vi "PlayConvolution.vi"(11 "File":T1) -> ()   [LabVIEW 2022 SP3]
uses:
  Curtin1_Label.ctl
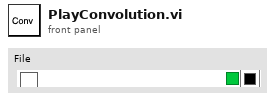
[diagram p1: front panel]
types:
  T1 = typedef "Curtin1_Label.ctl" = cluster{"Show?":bool, "Name":string, "Color":u32, "Path":path, "Show Notes":bool, "correlate":bool}
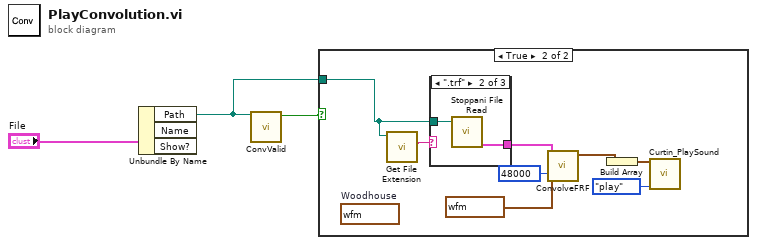
[diagram p0: block diagram]
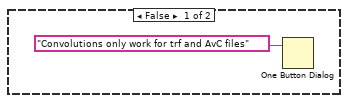
[diagram p2: hidden frame]
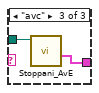
[diagram p4: hidden frame]
diagram:
  n1 = Unbundle By Name("File") -> ("Path"=w1:path)  [unwired: 2 out]
  n2 = call "ConvValid.vi"("Path"=w1) -> ("Valid"=w2:bool)  [unwired: 10 in]
  n3 = case shown="True" w2 {
    tunnel: w1 -> [_ w11]
    frame False {
      n4 = One Button Dialog(message="Convolutions only work for trf and AvC files" ("element")) -> ()  [unwired: 1 in, 1 out]
    }
    frame True {
      (unwired) waveform(dbl)[] [{"t0"=timestamp(0 s since 1904-01-01), "dt"=2.5e-05, "Y"=array[400000 elements]}]  # Woodhouse
      n5 = call <vilib>:"Get File Extension.vi"("file"=w11) -> ("lowercase file extension"=w12:string)  [unwired: 6 in, 4 out]
      n6 = case shown="\".trf\"" w12 {
        tunnel: [_ w14 w15] -> w10
        tunnel: w11 -> [_ w13 w16]
        frame Default {
        }
        frame ".trf" {
          n7 = call "Stoppani File Read.vi"("String in"=w13) -> ("Complex FRF"=w14:cluster{"t0":dbl, "dt":dbl, "Y":cdb[]})  [unwired: 2 in, 3 out]
        }
        frame "avc" {
          n8 = call "Stoppani_AvE.vi"("file (use dialog)"=w16) -> ("Complex FRF"=w15:cluster{"t0":dbl, "df":dbl, "Y":cdb[]})  [unwired: 7 in, 3 out]
        }
      }
      n9 = call "ConvolveFRF.vi"("musical piece"=waveform(dbl)[] [{"t0"=timestamp(0 s since 1904-01-01), "dt"=2.0833333333333333e-05, "Y"=array[288010 elements]}, {"t0"=timestamp(0 s since 1904-01-01), "dt"=2.0833333333333333e-05, "Y"=array[288010 elements]}], "Sampling rate"=u16 48000, "Complex FRF"=w10) -> ("Convolution"=w9:waveform(dbl))  [unwired: 5 in, 3 out]
      n10 = Build Array(w9) -> (w8:waveform(dbl)[])
      n11 = call "Curtin_PlaySound.vi"("Task"=enum16{"play", "save"}."play", "all waveforms"=w8) -> ()  [unwired: 9 in, 1 out]
    }
  }
